vi "Get Calibration Date.vi"(8 "error in (no error)":errorcluster, 11 "ICalibratable in":refnum<class "ICalibratable.lvclass">) -> (0 "error out":errorcluster, 2 "Time Stamp":timestamp format="%<%x %.3X>T", 3 "ICalibratable out":refnum<class "ICalibratable.lvclass">)   [LabVIEW 2023, in "ICalibratable.lvclass"]
uses:
  ICalibratable.lvclass
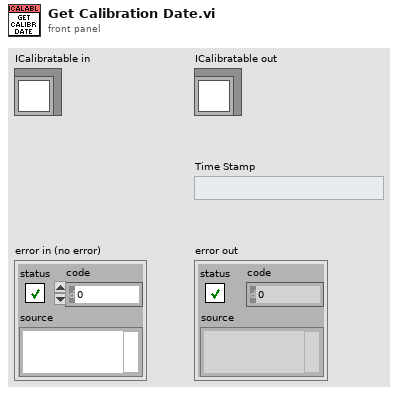
[diagram p1: front panel]
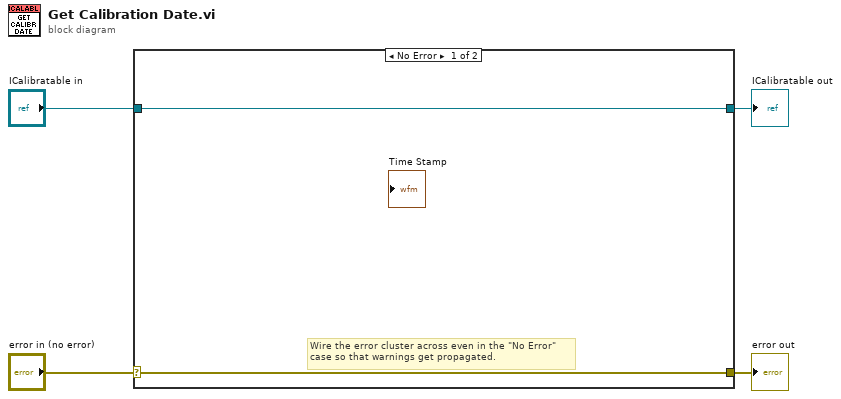
[diagram p0: block diagram]
diagram:
  n1 = case shown="No Error" "error in (no error)" {
    selector: "error in (no error)" -> [w5 w8]
    tunnel: [w5 w8] -> w3
    tunnel: [w6 w7] -> w1
    tunnel: "ICalibratable in" -> [w6 w7]
    frame No Error {
      # "Wire the error cluster across even in the \"No Error\"\ncase so that warnings get propagated."
    }
    frame Error {
    }
  }
  "error out" <- w3
  "ICalibratable out" <- w1
